vi "Shortest Distance Compressed.vi"(10 "Needed angle":dbl(knob) scale=0.0..360.0, 11 "Current Angle":dbl(knob) scale=0.0..360.0) -> (0 "Flip Motors?":bool=TRUE, 3 "Degrees to travel":dbl)   [LabVIEW 2013]
panel:
  # "Negative=Turn Left"
  # "Positive=Turn right"
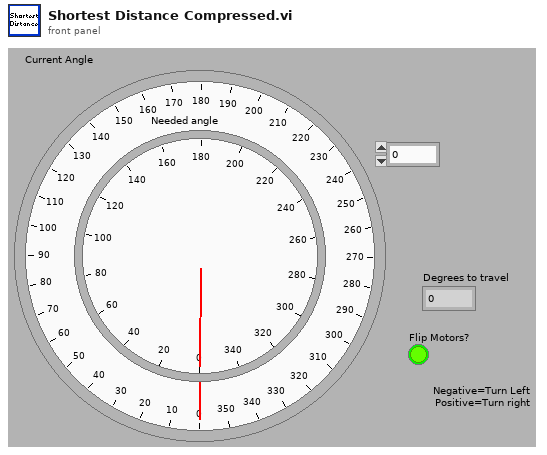
[diagram p1: front panel]
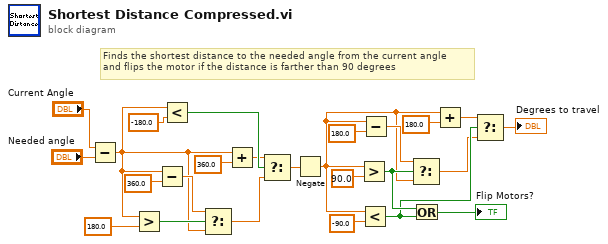
[diagram p0: block diagram]
diagram:
  # "Finds the shortest distance to the needed angle from the current angle\nand flips the motor if the distance is farther than 90 degrees"
  n1 = Subtract(x="Current Angle", y="Needed angle") -> (x-y=w16:dbl)
  n2 = Greater?(x=w16, y=180.0 ("x")) -> (0:w22:bool)
  n3 = Subtract(x=w16, y=360.0) -> (x-y=w20:dbl)
  n4 = Less?(x=w16, y=-180.0) -> (x < y?=w18:bool)
  n5 = Select(t=w20, s=w22, f=w16) -> (s? t:f=w14:dbl)
  n6 = Add(x=w16, y=360.0) -> (x+y=w15:dbl)
  n7 = Select(t=w15, s=w18, f=w14) -> (s? t:f=w13:dbl)
  n8 = Negate(x=w13) -> (-x=w2:dbl)
  n9 = Greater?(x=w2, y=90.0 ("x")) -> (0:w11:bool)
  n10 = Less?(x=w2, y=-90.0) -> (x < y?=w10:bool)
  n11 = Subtract(x=w2, y=180.0) -> (x-y=w8:dbl)
  n12 = Select(t=w8, s=w11, f=w2) -> (s? t:f=w9:dbl)
  n13 = Or(x=w11, y=w10) -> (x .or. y?=→"Flip Motors?":bool)
  n14 = Add(x=w2, y=180.0) -> (x+y=w6:dbl)
  n15 = Select(t=w6, s=w10, f=w9) -> (s? t:f=→"Degrees to travel":dbl)
